vi "target_new.vi"   [LabVIEW 2011]
uses:
  Output - Cluster.ctl
  Input - Cluster.ctl
  <vilib>/Platform/TimedLoop/XDataNode/timing_clust.ctl
  <vilib>/Platform/TimedLoop/XDataNode/nitl_modes.ctl
  <vilib>/Platform/TimedLoop/XDataNode/wakeup.ctl
  <vilib>/Platform/TimedLoop/XDataNode/XDataNode.xnode
  <vilib>/Platform/TimedLoop/XDataNode/XDNodeRunTimeDep.lvlib
panel:
  # "The Network Variable Engine and Variable Client Support must be installed on the RT target\nfor this application to function properly. If the Network Variable Engine is not supported on\nthe target (e.g.  FP-2000 with <32MB of RAM), open the project and move the variable library\nto My Computer in the project. Doing this will deploy the variables to localhost but\nwill still require that Variable Client Support be installed on the RT target."
types:
  T1 = typedef "Output - Cluster.ctl" = cluster{"DFS-1 [dl]":u64, "FS-3 [l]":dbl, "DFS-1 [l/min]":dbl, "DS-1 [bar]":dbl, "V-10 ZU":bool, "V-14 ZU":bool, "FS-1 [l]":dbl, "FS-2 [l]":dbl, "TS-4 [°C]":dbl, "HS-1":bool, "V-13 [%]":u8, "V-15 [%]":u8, "P-4 [%]":u8, "P-5 [%]":u8, "Dosierung":bool, "MR Max Füllstand":bool, "MR Min Füllstand":bool, "Dosiermenge [l]":sgl, "V-14 AUF":bool, "V-10 AUF":bool, "T-1 Max Füllstand":bool, "T-1 Min Füllstand":bool, "T-2 Max Füllstand":bool, "T-2 Min Füllstand":bool, "pHS-1 [pH]":dbl, "P-4 RUN":bool, "P-5 RUN ":bool, "V-33 AUF":bool, "V-33 ZU":bool, "V-34 AUF":bool, "V-34 ZU":bool, "P-4 ERR":bool, "P-5 ERR":bool, "TS-5 [°C]":dbl, "GZ-1 [dl]":u64, "TS-6 [°C]":dbl, "DS-3 [bar]":dbl}
  T2 = cluster{"Durchflussregelung":dbl, "Temperaturregelung":bool, "STOP":bool, "Zirkulation":u64, "Dosierung Zeit":u64}
  T3 = typedef "XDNodeRunTimeDep.lvlib/timing_clust.ctl" = cluster{"Expected End [f-1]":u64, "Actual End [f-1]":u64, "Finished Late? [f-1]":bool, "Expected End [i-1]":u64, "Actual End [i-1]":u64, "Finished Late? [i-1]":bool, "Expected Start [i]":u64, "Actual Start [i]":u64, "Expected Start [f]":u64, "Actual Start [f]":u64, "Source Name":string, "Structure Name":string, "Period":i64, "Deadline":i64, "Offset":i64, "Start":i64, "Priority":i32, "Timeout":i32, "Mode":T4, "Wakeup Reason":T5, "Error":errorcluster, "Source Type":string, "Secondary Source Type":string, "Global End Time":u64, "Global Start Time":u64, "Frame Duration":u64, "Iteration Duration":u64, "Assigned CPU":i32, "I/O Scan Engine Mode":u32}
  T4 = typedef "XDNodeRunTimeDep.lvlib/nitl_modes.ctl" = enum32{"No Change", "Process missed periods, maintain original phase", "Discard missed periods, maintain original phase", "Process missed periods, ignore original phase", "Discard missed periods, ignore original phase"}
  T5 = typedef "XDNodeRunTimeDep.lvlib/wakeup.ctl" = enum32{"Normal", "Aborted", "Asynchronous wakeup", "Timing source error", "Timed loop error", "Timeout"}
  T6 = typedef "Input - Cluster.ctl" = cluster{"V-13 [%]":u8, "V-15 [%]":u8, "Log-Target":bool, "P-4":bool, "P-4 Drehzahl [%]":u8, "Temperaturregelung":bool, "Überdruckregelung":bool, "Füllstandsregulierung":bool, "V-10":bool, "Log-Host":bool, "V-14":bool, "P-5":bool, "P-5 Drehzahl [%]":u8, "HS-1":bool, "Füllstand  P":sgl, "Füllstand I":sgl, "Füllstand D":sgl, "Füllstand Soll [l]":sgl, "Druck  P":sgl, "Druck I":sgl, "Druck D":sgl, "Druck Soll [bar]":sgl, "Temp Soll [°C]":sgl, "Dosierung":bool, "Dosiermenge [l]":sgl, "Dosiergeschw. [l/min]":sgl, "Tank":bool, "Hysterese [°C]":sgl, "MR Füllstandsüberwachung":bool, "Tank Füllstandsüberwachung":bool, "Log Target [ms]":u32, "Log Host [s]":u32, "P-5 EIN [min]":u8, "P-5 AUS [min]":u8, "Zirkulation":bool, "V-33":bool, "V-34":bool}
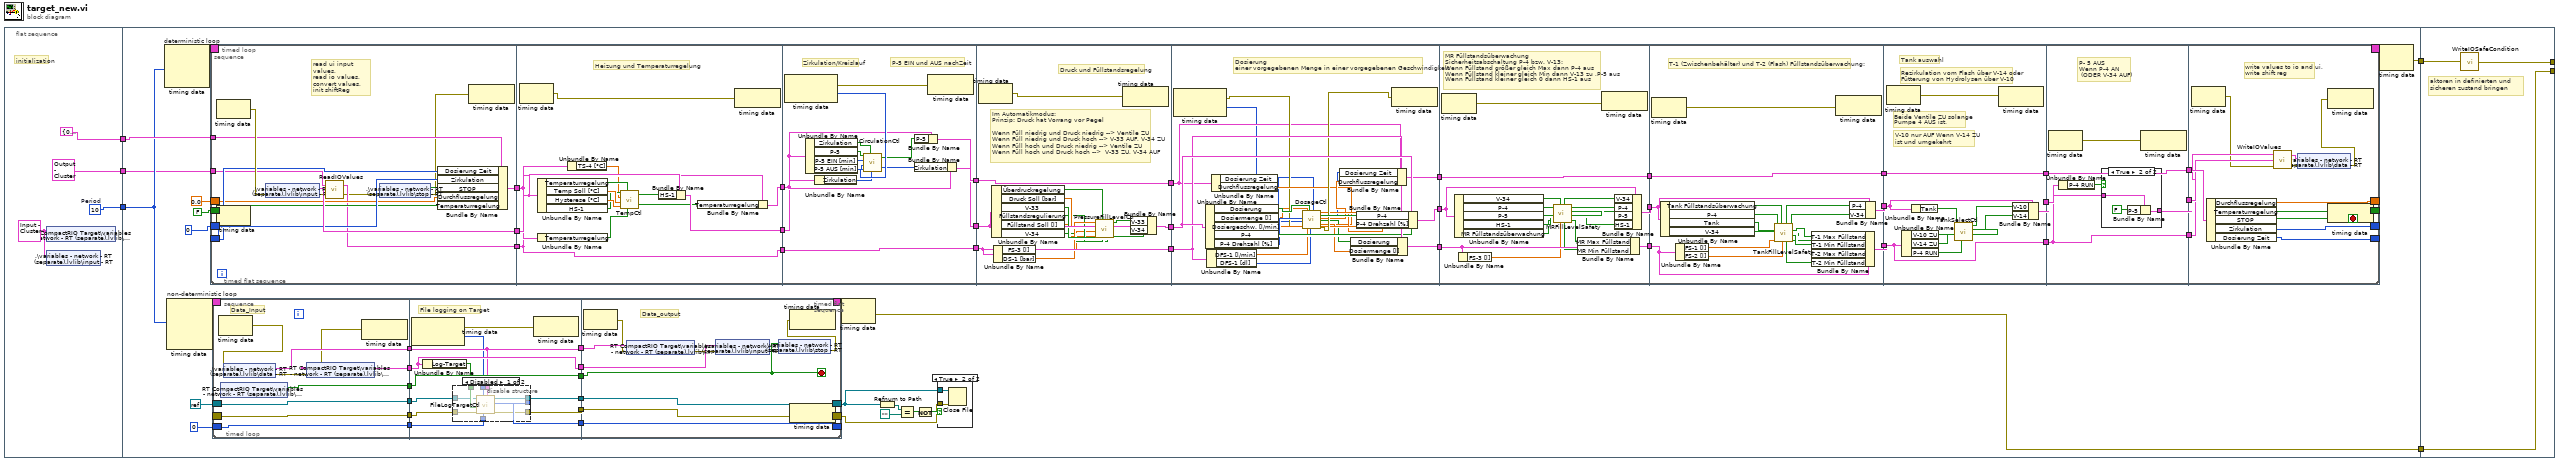
[diagram p0: block diagram]
diagram:
  n1 = flat-sequence {
    tunnel: [T2 {"Durchflussregelung"=0.0, "Temperaturregelung"=FALSE, "STOP"=FALSE, "Zirkulation"=0, "Dosierung Zeit"=0} ("rt_vars")] -> w5
    tunnel: [w7] -> w4
    tunnel: [T1 {"DFS-1 [dl]"=0, "FS-3 [l]"=0.0, "DFS-1 [l/min]"=0.0, "DS-1 [bar]"=0.0, "V-10 ZU"=FALSE, "V-14 ZU"=FALSE, "FS-1 [l]"=0.0, "FS-2 [l]"=0.0, "TS-4 [°C]"=0.0, "HS-1"=FALSE, "V-13 [%]"=0, "V-15 [%]"=0, "P-4 [%]"=0, "P-5 [%]"=0, "Dosierung"=FALSE, "MR Max Füllstand"=FALSE, "MR Min Füllstand"=FALSE, "Dosiermenge [l]"=0.0, "V-14 AUF"=FALSE, "V-10 AUF"=FALSE, "T-1 Max Füllstand"=FALSE, "T-1 Min Füllstand"=FALSE, "T-2 Max Füllstand"=FALSE, "T-2 Min Füllstand"=FALSE, "pHS-1 [pH]"=0.0, "P-4 RUN"=FALSE, "P-5 RUN "=FALSE, "V-33 AUF"=FALSE, "V-33 ZU"=FALSE, "V-34 AUF"=FALSE, "V-34 ZU"=FALSE, "P-4 ERR"=FALSE, "P-5 ERR"=FALSE, "TS-5 [°C]"=0.0, "GZ-1 [dl]"=0, "TS-6 [°C]"=0.0, "DS-3 [bar]"=0.0} ("Output - Cluster")] -> w3
    tunnel: w5 -> [w16]
    tunnel: w4 -> [w15]
    tunnel: w3 -> [w14]
    tunnel: [w13] -> w2
    tunnel: [w12] -> w1
    tunnel: w2 -> [w375]
    tunnel: w1 -> [w377]
    tunnel: [w376] -> _
    tunnel: [w375] -> _
    frame #0 {
      w7 = i64 10  # Period
      w9 = T6 {"V-13 [%]"=0, "V-15 [%]"=0, "Log-Target"=FALSE, "P-4"=FALSE, "P-4 Drehzahl [%]"=0, "Temperaturregelung"=FALSE, "Überdruckregelung"=FALSE, "Füllstandsregulierung"=FALSE, "V-10"=FALSE, "Log-Host"=FALSE, "V-14"=FALSE, "P-5"=FALSE, "P-5 Drehzahl [%]"=0, "HS-1"=FALSE, "Füllstand  P"=0.0, "Füllstand I"=0.0, "Füllstand D"=0.0, "Füllstand Soll [l]"=0.0, "Druck  P"=0.0, "Druck I"=0.0, "Druck D"=0.0, "Druck Soll [bar]"=0.0, "Temp Soll [°C]"=0.0, "Dosierung"=FALSE, "Dosiermenge [l]"=0.0, "Dosiergeschw. [l/min]"=0.0, "Tank"=FALSE, "Hysterese [°C]"=0.0, "MR Füllstandsüberwachung"=FALSE, "Tank Füllstandsüberwachung"=FALSE, "Log Target [ms]"=0, "Log Host [s]"=0, "P-5 EIN [min]"=0, "P-5 AUS [min]"=0, "Zirkulation"=FALSE, "V-33"=FALSE, "V-34"=FALSE} ("Input - Cluster")
      # "initialization"
      n2 = shared-variable "RT CompactRIO Target\\variables - network - RT (separate).lvlib\\input - network"(w9) -> ()  [unwired: 1 in, 1 out]
      n3 = shared-variable ".\\variables - network - RT (separate).lvlib\\input - RT"(w9) -> ()  [unwired: 1 in, 1 out]
    }
    frame #1 {
      w11 = u64 0
      n4 = node-c288 ("Input Node")(w15) -> (w29:T3)  [unwired: 2 in]
      n5 = node-c288 ("Input Node")(w15) -> (w27:T3)  [unwired: 3 in]
      n6 = timed-loop "deterministic loop" {
        timing: w29 -> [_]
        timing-out: [_] -> w28
        shift-right: [w128] -> _
        shift-left: 0.0 -> [w127]
        shift-right: [w126] -> _
        shift-left: FALSE ("Temperaturregelung") -> [w124]
        tunnel: w16 -> [w125]
        tunnel: w14 -> [w123]
        shift-right: [w122] -> _
        shift-left: w11 -> [w121]
        shift-right: [w120] -> _
        shift-left: w11 -> [w119]
        stop <- w358 stop-if-true
        n7 = timed-sequence {
          timing: _ -> [_]
          timing-out: _ -> [_]
          tunnel: [w163] -> w128
          tunnel: w127 -> [w162]
          tunnel: [w159] -> w126
          tunnel: w125 -> [w158]
          tunnel: w124 -> [w156]
          tunnel: w123 -> [w151]
          tunnel: [w138] -> w122
          tunnel: w121 -> [w137]
          tunnel: [w130] -> w120
          tunnel: w119 -> [w129]
          n8 = timed-flat-sequence {
            tunnel: [w179] -> w161
            tunnel: [w169] -> w160
            tunnel: w162 -> [w172]
            tunnel: w158 -> [w177]
            tunnel: [w176] -> w157
            tunnel: w156 -> [w171]
            tunnel: w151 -> [w170]
            tunnel: w137 -> [w175]
            tunnel: w129 -> [w174]
            tunnel: w161 -> [w194]
            tunnel: w160 -> [w186]
            tunnel: [w186] -> w144
            tunnel: w157 -> [w190]
            tunnel: [w191] -> w142
            tunnel: [w193] -> w140
            tunnel: w144 -> [w216]
            tunnel: [w216] -> w143
            tunnel: w142 -> [w209]
            tunnel: [w210] -> w141
            tunnel: w140 -> [w207]
            tunnel: [w208] -> w139
            tunnel: [w236] -> w165
            tunnel: w143 -> [w234]
            tunnel: [w234] -> w164
            tunnel: w141 -> [w238]
            tunnel: [w238] -> w155
            tunnel: w139 -> [w235]
            tunnel: w165 -> [w267]
            tunnel: [w265] -> w150
            tunnel: w164 -> [w266]
            tunnel: [w260] -> w149
            tunnel: w155 -> [w252]
            tunnel: [w256] -> w148
            tunnel: w150 -> [w280]
            tunnel: [w279] -> w154
            tunnel: w149 -> [w289]
            tunnel: [w288] -> w153
            tunnel: w148 -> [w291]
            tunnel: [w291] -> w152
            tunnel: w154 -> [w301]
            tunnel: [w302] -> w147
            tunnel: w153 -> [w312]
            tunnel: [w311] -> w146
            tunnel: w152 -> [w314]
            tunnel: [w314] -> w145
            tunnel: w147 -> [w322]
            tunnel: [w323] -> w136
            tunnel: w146 -> [w327]
            tunnel: [w327] -> w134
            tunnel: w145 -> [w330]
            tunnel: [w330] -> w132
            tunnel: w136 -> [w339]
            tunnel: [w338] -> w135
            tunnel: w134 -> [w337]
            tunnel: [w337] -> w133
            tunnel: w132 -> [w341]
            tunnel: [w341] -> w131
            tunnel: w135 -> [w355]
            tunnel: w133 -> [w354]
            tunnel: [w359] -> w163
            tunnel: [w360] -> w159
            tunnel: w131 -> [w361]
            tunnel: [w357] -> w138
            tunnel: [w356] -> w130
            frame #0 {
              # "read ui input values,\nread io values,\nconvert values,\ninit shiftReg"
              n9 = node-c288 ("Output Node")() -> (w178:errorcluster)  [unwired: 1 in]
              n10 = shared-variable ".\\variables - network - RT (separate).lvlib\\input - RT"(error in=w178) -> (w179:T6, error out=w168:errorcluster)
              n11 = call "ReadIOValues.vi"("error in"=w168, "Output - Cluster"=w170) -> ("error out"=w167:errorcluster, "output cluster"=w169:T1)
              n12 = shared-variable ".\\variables - network - RT (separate).lvlib\\stop - RT"(error in=w167) -> (w173:bool, error out=w166:errorcluster)
              n13 = Bundle By Name(cluster=w177, "Dosierung Zeit"=w174, "Zirkulation"=w175, "STOP"=w173, "Durchflussregelung"=w172, "Temperaturregelung"=w171) -> (w176:T2)
              n14 = node-c288 ("Input Node")(w166) -> ()  [unwired: 1 out]
            }
            frame #1 {
              # "Heizung und Temperaturregelung"
              n15 = node-c288() -> (w198:errorcluster)  [unwired: 1 in]
              n16 = Unbundle By Name(w194) -> ("Temperaturregelung"=w197:bool, "Temp Soll [°C]"=w196:sgl, "Hysterese [°C]"=w195:sgl, "HS-1"=w187:bool)
              n17 = Unbundle By Name(w190) -> ("Temperaturregelung"=w189:bool)
              n18 = Unbundle By Name(w186) -> ("TS-4 [°C]"=w185:dbl)
              n19 = call "TempCtl.vi"("shiftReg"=w189, "enable"=w197, "Hysterese"=w195, "Soll"=w196, "IST"=w185, "heating"=w187) -> ("shiftReg"=w188:bool, "heating"=w192:bool)
              n20 = Bundle By Name(cluster=w194, "HS-1"=w192) -> (w193:T6)
              n21 = Bundle By Name(cluster=w190, "Temperaturregelung"=w188) -> (w191:T2)
              n22 = node-c288(w198) -> ()  [unwired: 1 out]
            }
            frame #2 {
              # "P-5 EIN und AUS nachZeit"
              # "Zirkulation/Kreislauf"
              n23 = node-c288() -> (w217:errorcluster, w215:i64)  [unwired: 1 in]
              n24 = Unbundle By Name(w207) -> ("Zirkulation"=w212:bool, "P-5"=w211:bool, "P-5 EIN [min]"=w214:u8, "P-5 AUS [min]"=w213:u8)
              n25 = Unbundle By Name(w209) -> ("Zirkulation"=w204:u64)
              n26 = call "CirculationCtl.vi"("shiftReg[ms]"=w204, "enable"=w212, "Actual Start [ms]"=w215, "OffTime [min]"=w213, "OnTime [min]"=w214, "Pump"=w211) -> ("shiftReg[ms]"=w205:u64, "Pump"=w206:bool)
              n27 = Bundle By Name(cluster=w207, "P-5"=w206) -> (w208:T6)
              n28 = Bundle By Name(cluster=w209, "Zirkulation"=w205) -> (w210:T2)
              n29 = node-c288(w217) -> ()  [unwired: 1 out]
            }
            frame #3 {
              # "Im Automatikmodus:\nPrinzip: Druck hat Vorrang vor Pegel\n\nWenn Füll niedrig und Druck niedrig --> Ventile ZU\nWenn Füll niedrig und Druck hoch --> V-33 AUF, V-34 ZU\nWenn Füll hoch und Druck niedrig --> Ventile ZU\nWenn Füll hoch und Druck hoch -->  V-33 ZU, V-34 AUF"
              # "Druck und Füllstandsregelung"
              n30 = node-c288() -> (w237:errorcluster)  [unwired: 1 in]
              n31 = Unbundle By Name(w235) -> ("Überdruckregelung"=w233:bool, "Druck Soll [bar]"=w231:sgl, "V-33"=w232:bool, "Füllstandsregulierung"=w229:bool, "Füllstand Soll [l]"=w227:sgl, "V-34"=w228:bool)
              n32 = Unbundle By Name(w234) -> ("FS-3 [l]"=w226:dbl, "DS-1 [bar]"=w230:dbl)
              n33 = call "PressureFillLevelCtl.vi"("LiquidValve"=w228, "GasValve"=w232, "FillLevelCtl"=w229, "PressureCtl"=w233, "V_setpoint"=w227, "V_value"=w226, "P_setpoint"=w231, "P_value"=w230) -> ("LiquidValve"=w224:bool, "GasValve"=w225:bool)  [unwired: 2 in]
              n34 = node-c288(w237) -> ()  [unwired: 1 out]
              n35 = Bundle By Name(cluster=w235, "V-33"=w225, "V-34"=w224) -> (w236:T6)
            }
            frame #4 {
              # "Dosierung \neiner vorgegebenen Menge in einer vorgegebenen Geschwindigkeit"
              n36 = node-c288() -> (w253:errorcluster, w247:i64)  [unwired: 1 in]
              n37 = Unbundle By Name(w267) -> ("Dosierung"=w258:bool, "Dosiermenge [l]"=w244:sgl, "Dosiergeschw. [l/min]"=w261:sgl, "P-4"=w264:bool, "P-4 Drehzahl [%]"=w263:u8)
              n38 = Unbundle By Name(w266) -> ("DFS-1 [l/min]"=w249:dbl, "DFS-1 [dl]"=w250:u64)
              n39 = Unbundle By Name(w252) -> ("Dosierung Zeit"=w248:u64, "Durchflussregelung"=w254:dbl)
              n40 = call "DosageCtl.vi"("setpoint volume flow [l/min]"=w261, "pump"=w264, "value speed [%]"=w263, "shiftReg int"=w248, "shiftReg dbl"=w254, "error in (no error)"=w253, "setpoint volume [l]"=w244, "value volume flow [l/min]"=w249, "enable"=w258, "value volume [dl]"=w250, "Actual Start [f]"=w247) -> ("pump"=w251:bool, "speed [%]"=w259:dbl, "shiftReg int"=w246:u64, "shiftreg dbl"=w255:dbl, "enable"=w245:bool, "volume[l]"=w257:dbl, "error out"=w262:errorcluster)  [unwired: 2 in]
              n41 = Bundle By Name(cluster=w252, "Dosierung Zeit"=w246, "Durchflussregelung"=w255) -> (w256:T2)
              n42 = Bundle By Name(cluster=w266, "Dosierung"=w245, "Dosiermenge [l]"=w257) -> (w260:T1)
              n43 = Bundle By Name(cluster=w267, "P-4"=w251, "P-4 Drehzahl [%]"=w259) -> (w265:T6)
              n44 = node-c288(w262) -> ()  [unwired: 1 out]
            }
            frame #5 {
              # "MR Füllstandsüberwachung\nSicherheitsabschaltung P-4 bzw. V-13:\nWenn Füllstand größer gleich Max dann P-4 aus\nWenn Füllstand kleiner gleich Min dann V-13 zu ,P-5 aus\nWenn Füllstand kleiner gleich 0 dann HS-1 aus"
              n45 = node-c288() -> (w290:errorcluster)  [unwired: 1 in]
              n46 = Unbundle By Name(w280) -> ("V-34"=w284:bool, "P-4"=w283:bool, "P-5"=w282:bool, "HS-1"=w281:bool, "MR Füllstandsüberwachung"=w274:bool)
              n47 = Unbundle By Name(w289) -> ("FS-3 [l]"=w285:dbl)
              n48 = call "MRFillLevelSafety.vi"("fill level [l]"=w285, "Valve"=w284, "enable"=w274, "Heating"=w281, "Circulation"=w282, "Pump"=w283) -> ("max level"=w287:bool, "Heating"=w275:bool, "Circulation"=w276:bool, "Pump"=w277:bool, "min level"=w286:bool, "Valve"=w278:bool)
              n49 = Bundle By Name(cluster=w289, "MR Max Füllstand"=w287, "MR Min Füllstand"=w286) -> (w288:T1)
              n50 = node-c288(w290) -> ()  [unwired: 1 out]
              n51 = Bundle By Name(cluster=w280, "V-34"=w278, "P-4"=w277, "P-5"=w276, "HS-1"=w275) -> (w279:T6)
            }
            frame #6 {
              # "T-1 (Zwischenbehälter) und T-2 (Flash) Füllstandsüberwachung:"
              n52 = node-c288() -> (w313:errorcluster)  [unwired: 1 in]
              n53 = Unbundle By Name(w301) -> ("Tank Füllstandsüberwachung"=w297:bool, "P-4"=w300:bool, "Tank"=w298:bool, "V-34"=w299:bool)
              n54 = Unbundle By Name(w312) -> ("FS-1 [l]"=w306:dbl, "FS-2 [l]"=w308:dbl)
              n55 = call "TankFillLevelSafety.vi"("fill level t-2"=w308, "enable"=w297, "fill level t-1"=w306, "valve"=w299, "tank"=w298, "pump"=w300) -> ("max level t-2"=w307:bool, "min level t-1"=w310:bool, "max level t-1"=w305:bool, "valve"=w303:bool, "min level t-2"=w309:bool, "pump"=w304:bool)
              n56 = Bundle By Name(cluster=w312, "T-1 Max Füllstand"=w305, "T-1 Min Füllstand"=w310, "T-2 Max Füllstand"=w307, "T-2 Min Füllstand"=w309) -> (w311:T1)
              n57 = node-c288(w313) -> ()  [unwired: 1 out]
              n58 = Bundle By Name(cluster=w301, "P-4"=w304, "V-34"=w303) -> (w302:T6)
            }
            frame #7 {
              # "V-10 nur AUF Wenn V-14 ZU\nist und umgekehrt"
              # "Beide Ventile ZU solange \nPumpe 4 AUS ist."
              # "Rezirkulation vom Flash über V-14 oder \nFütterung von Hydrolysen über V-10"
              # "Tank auswahl"
              n59 = node-c288() -> (w328:errorcluster)  [unwired: 1 in]
              n60 = Unbundle By Name(w327) -> ("V-10 ZU"=w325:bool, "V-14 ZU"=w326:bool, "P-4 RUN"=w324:bool)
              n61 = Unbundle By Name(w322) -> ("Tank"=w329:bool)
              n62 = call "TankSelectCtl.vi"("pump"=w324, "valve t-2 close"=w326, "valve t-1 close"=w325, "Tank"=w329) -> ("valve t-2"=w320:bool, "valve t-1"=w321:bool)  [unwired: 6 in]
              n63 = node-c288(w328) -> ()  [unwired: 1 out]
              n64 = Bundle By Name(cluster=w322, "V-10"=w321, "V-14"=w320) -> (w323:T6)
            }
            frame #8 {
              # "P- 5 AUS \nWenn P-4 AN\n (ODER V-34 AUF)"
              n65 = node-c288() -> (w340:errorcluster)  [unwired: 1 in]
              n66 = Unbundle By Name(w337) -> ("P-4 RUN"=w336:bool)
              n67 = case shown="True" w336 {
                tunnel: w339 -> [w342 w345]
                tunnel: [w342 w344] -> w338
                frame False {
                }
                frame True {
                  n68 = Bundle By Name(cluster=w345, "P-5"=FALSE) -> (w344:T6)
                }
              }
              n69 = node-c288(w340) -> ()  [unwired: 1 out]
            }
            frame #9 {
              # "write values to io and ui,\nwrite shift reg"
              n70 = node-c288() -> (w352:errorcluster)  [unwired: 1 in]
              n71 = Unbundle By Name(w361) -> ("Durchflussregelung"=w359:dbl, "Temperaturregelung"=w360:bool, "STOP"=w358:bool, "Zirkulation"=w357:u64, "Dosierung Zeit"=w356:u64)
              n72 = call "WriteIOValues.vi"("error in"=w352, "Output - Cluster"=w354, "input cluster"=w355) -> ("error out"=w351:errorcluster, "output cluster"=w353:T1)
              n73 = shared-variable ".\\variables - network - RT (separate).lvlib\\data - RT"(w353, error in=w351) -> (error out=w362:errorcluster)
              n74 = node-c288(w362) -> ()  [unwired: 1 out]
            }
          }
        }
        n75 = node-c288() -> ()  [unwired: 1 in, 1 out]
        n76 = node-c288() -> ()  [unwired: 1 in, 1 out]
      }
      n77 = timed-loop "non-deterministic loop" {
        timing: w27 -> [_]
        timing-out: [_] -> w26
        shift-right: [w37] -> _
        shift-left: i64 0 ("Actual Start [f]") -> [w36]
        shift-right: [w35] -> w20
        shift-left: refnum<k0> refnum -> [w34]
        shift-right: [w33] -> w21
        shift-left: _ -> [w32]
        stop <- w104 stop-if-true
        n78 = timed-sequence {
          timing: _ -> [_]
          timing-out: _ -> [_]
          tunnel: [w46] -> w37
          tunnel: w36 -> [w44]
          tunnel: [w43] -> w35
          tunnel: w34 -> [w41]
          tunnel: [w40] -> w33
          tunnel: w32 -> [w38]
          n79 = timed-flat-sequence {
            tunnel: [w63] -> w55
            tunnel: [w64] -> w54
            tunnel: [w62] -> w49
            tunnel: [w58] -> w45
            tunnel: w44 -> [w58]
            tunnel: [w57] -> w42
            tunnel: w41 -> [w57]
            tunnel: [w56] -> w39
            tunnel: w38 -> [w56]
            tunnel: w55 -> [w80]
            tunnel: w54 -> [w78]
            tunnel: [w74] -> w53
            tunnel: [w75] -> w52
            tunnel: [w80] -> w51
            tunnel: [w79] -> w50
            tunnel: w49 -> [w79]
            tunnel: [w78] -> w48
            tunnel: [w73] -> w47
            tunnel: w45 -> [w76]
            tunnel: w42 -> [w71]
            tunnel: w39 -> [w70]
            tunnel: w53 -> [w106]
            tunnel: w52 -> [w105]
            tunnel: w51 -> [w104]
            tunnel: w50 -> [w103]
            tunnel: w48 -> [w102]
            tunnel: w47 -> [w97]
            tunnel: [w97] -> w46
            tunnel: [w105] -> w43
            tunnel: [w106] -> w40
            frame #0 {
              # "Data_Input"
              n80 = node-c288() -> (w61:errorcluster)  [unwired: 1 in]
              n81 = shared-variable "RT CompactRIO Target\\variables - network - RT (separate).lvlib\\stop - network"() -> (w63:bool)  [unwired: 1 in, 1 out]
              n82 = shared-variable ".\\variables - network - RT (separate).lvlib\\data - RT"(error in=w61) -> (w64:T1, error out=w60:errorcluster)
              n83 = shared-variable "RT CompactRIO Target\\variables - network - RT (separate).lvlib\\input - network"(error in=w60) -> (w62:T6, error out=w59:errorcluster)
              n84 = node-c288(w59) -> ()  [unwired: 1 out]
            }
            frame #1 {
              # "File logging on Target"
              n85 = node-c288() -> (w81:errorcluster, w77:i64)  [unwired: 1 in]
              n86 = Unbundle By Name(w79) -> ("Log-Target"=w72:bool)
              n87 = disable-structure shown="Disabled" {
                disable-tunnel: w78 -> [w90 _]
                disable-tunnel: w77 -> [w89 _]
                disable-tunnel: w76 -> [w88 _]
                disable-tunnel: [w87 _] -> w75
                disable-tunnel: [w86 _] -> w74
                disable-tunnel: [w85 _] -> w73
                disable-tunnel: w72 -> [w84 _]
                disable-tunnel: w71 -> [w83 _]
                disable-tunnel: w70 -> [w82 _]
                frame Disabled {
                  n88 = call "FileLogTargetCtl.vi"("Actual Start [f] in"=w88, "Actual Start [f] 3"=w89, "error in (no error)"=w82, "Log-Target"=w84, "Output - Cluster"=w90, "Byte Stream File in"=w83) -> ("error out"=w86:errorcluster, "Actual Start [f] out"=w85:i64, "Byte Stream File out"=w87:refnum<file>)  [unwired: 3 in]
                }
                frame Enabled {
                }
              }
              n89 = node-c288(w81) -> ()  [unwired: 1 out]
            }
            frame #2 {
              # "Data_output"
              n90 = node-c288() -> (w101:errorcluster)  [unwired: 1 in]
              n91 = shared-variable "RT CompactRIO Target\\variables - network - RT (separate).lvlib\\data - network"(w102, error in=w101) -> (error out=w100:errorcluster)
              n92 = shared-variable ".\\variables - network - RT (separate).lvlib\\input - RT"(w103, error in=w100) -> (error out=w99:errorcluster)
              n93 = shared-variable ".\\variables - network - RT (separate).lvlib\\stop - RT"(w104, error in=w99) -> (error out=w98:errorcluster)
              n94 = node-c288(w98) -> ()  [unwired: 1 out]
            }
          }
        }
        n95 = node-c288() -> ()  [unwired: 1 in, 1 out]
        n96 = node-c288() -> ()  [unwired: 1 in, 1 out]
      }
      n97 = node-c288 ("Output Node")(w26) -> (w13:errorcluster)
      n98 = Refnum to Path(1:w20) -> (0:w19:path)
      n99 = Equal?(x=w19, y=path "") -> (x = y?=w23:bool)
      n100 = Not(x=w23) -> (.not. x?=w22:bool)
      n101 = case shown="True" w22 {
        tunnel: w20 -> [_ w31]
        tunnel: w21 -> [_ w30]
        frame False {
        }
        frame True {
          n102 = Close File(refnum=w31, error in=w30) -> ()  [unwired: 2 out]
        }
      }
      n103 = node-c288 ("Output Node")(w28) -> (w12:errorcluster)
    }
    frame #2 {
      # "aktoren in definierten und sicheren zustand bringen"
      n104 = call "WriteIOSafeCondition.vi"("error in"=w377) -> ("error out"=w376:errorcluster)
    }
  }
